vi "Selection_with_Search.vi"(1 "Selected Channel Names":string[](array[string]), 2 "Search String":string, 3 "All Channel Names":string[](array[string])) -> (0 "Item Names":string[](array[string]))   [LabVIEW 2010]
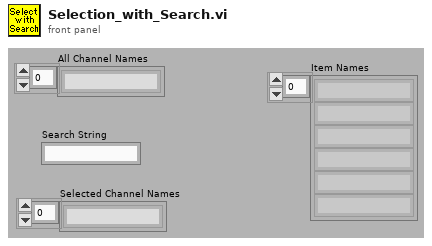
[diagram p1: front panel]
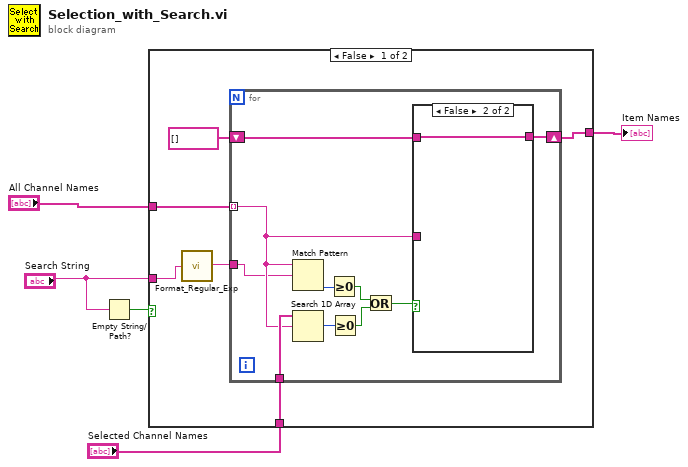
[diagram p0: block diagram]
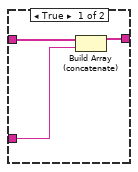
[diagram p2: hidden frame]
diagram:
  n1 = Empty String/Path?(string/path="Search String") -> (empty?=w3:bool)
  n2 = case shown="False" w3 {
    tunnel: "Search String" -> [w7 _]
    tunnel: "All Channel Names" -> [w11 w26]
    tunnel: [w9 w26] -> w4
    tunnel: "Selected Channel Names" -> [w8 _]
    frame False {
      n3 = call "Format_Regular_Exp.vi"("Regular expression"=w7) -> ("Case Insensitive for html"=w6:string)
      n4 = for {
        shift-right: [w20] -> w9
        shift-left: string[] [] -> [w21]
        tunnel: w6 -> [w12]
        tunnel: w11 -> [w13] mode=indexing
        tunnel: w8 -> [w19]
        n5 = Match Pattern(string=w13, regular expression=w12) -> (offset past match=w18:i32)  [unwired: 4 out]
        n6 = Search 1D Array(1D array=w19, element=w13) -> (index of element=w17:i32)  [unwired: 1 out]
        n7 = Greater Or Equal To 0?(x=w18) -> (x >= 0?=w15:bool)
        n8 = Greater Or Equal To 0?(x=w17) -> (x >= 0?=w16:bool)
        n9 = Or(x=w15, y=w16) -> (x .or. y?=w14:bool)
        n10 = case shown="False" w14 {
          tunnel: w21 -> [w24 w25]
          tunnel: [w23 w25] -> w20
          tunnel: w13 -> [w22 _]
          frame True {
            n11 = Build Array (concatenate)(w24, w22) -> (w23:string[])
          }
          frame False {
          }
        }
      }
    }
    frame True {
    }
  }
  "Item Names" <- w4
